vi "CT-Sweep One Component.vi"(0 "Phase In":dbl=100000.0, 5 "Last Freq (Hz)":dbl=100000.0, 7 "New Freq (Hz)":dbl=100000.0, 9 "dt (s)":dbl=100000.0, 11 "Npts":i32, 13 "randomize phase":bool) -> (4 "Phase Out":dbl, 8 "Y":dbl[](array[numeric]))   [LabVIEW 2015]
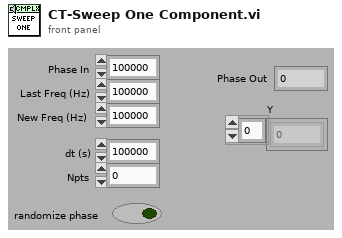
[diagram p1: front panel]
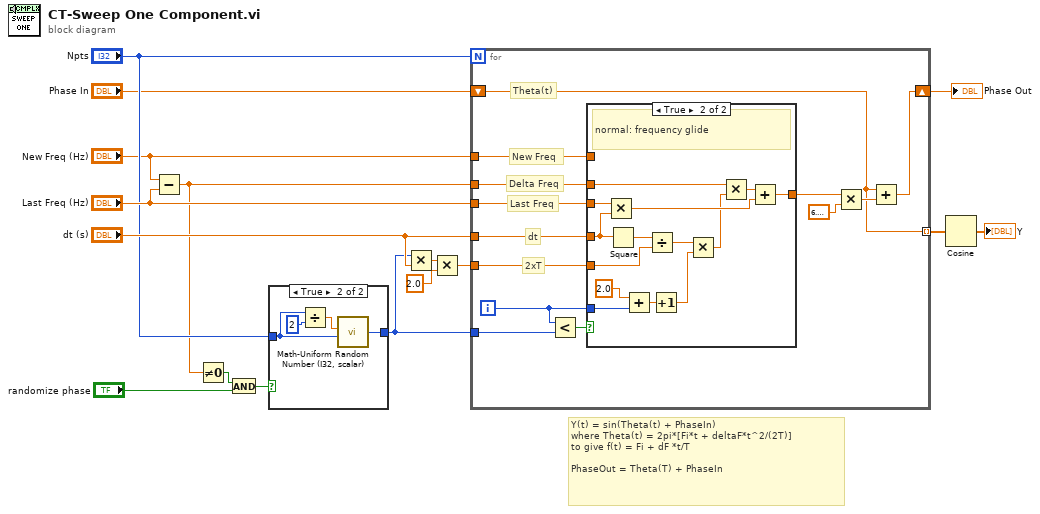
[diagram p0: block diagram]
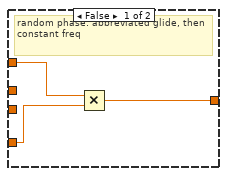
[diagram p3: hidden frame]
diagram:
  # "Y(t) = sin(Theta(t) + PhaseIn)\nwhere Theta(t) = 2pi*[Fi*t + deltaF*t^2/(2T)]\nto give f(t) = Fi + dF *t/T \n\nPhaseOut = Theta(T) + PhaseIn"
  n1 = Subtract(x="New Freq (Hz)", y="Last Freq (Hz)") -> (x-y=w6:dbl)
  n2 = Not Equal To 0?(x=w6) -> (x != 0?=w7:bool)
  n3 = And(x=w7, y="randomize phase") -> (x .and. y?=w3:bool)
  n4 = case shown="True" w3 {
    tunnel: "Npts" -> [w17 w20]
    tunnel: [w17 w18] -> w8
    frame False {
    }
    frame True {
      n5 = Divide(x=w20, y=2) -> (x/y=w19:dbl)
      n6 = call "Math-Uniform Random Number (I32, scalar).vi"("Ymax"=w20, "Ymin"=w19) -> ("Random Int"=w18:i32)  [unwired: 4 in]
    }
  }
  n7 = Multiply(x=w8, y="dt (s)") -> (x*y=w15:dbl)
  n8 = Multiply(x=w15, y=2.0) -> (x*y=w13:dbl)
  n9 = for {
    N: "Npts" -> [_]
    tunnel: "dt (s)" -> [w33]
    shift-right: [w29] -> w1
    shift-left: "Phase In" -> [w22]
    tunnel: "Last Freq (Hz)" -> [w34]
    tunnel: w13 -> [w27]
    tunnel: w6 -> [w28]
    tunnel: [w22] -> w4 mode=indexing
    tunnel: w8 -> [w25]
    tunnel: "New Freq (Hz)" -> [w24]
    i -> [w26]
    # "New Freq"
    # "dt"
    # "2xT"
    # "Theta(t)"
    # "Last Freq"
    # "Delta Freq"
    n10 = Less?(x=w26, y=w25) -> (x < y?=w23:bool)
    n11 = case shown="True" w23 {
      tunnel: w34 -> [_ w51]
      tunnel: w33 -> [w37 w50]
      tunnel: [w36 w45] -> w32
      tunnel: w28 -> [_ w44]
      tunnel: w27 -> [_ w43]
      tunnel: w26 -> [_ w41]
      tunnel: w24 -> [w35 _]
      frame False {
        # "random phase: abbreviated glide, then constant freq"
        n12 = Multiply(x=w35, y=w37) -> (x*y=w36:dbl)
      }
      frame True {
        # "normal: frequency glide"
        n13 = Multiply(x=w51, y=w50) -> (x*y=w46:dbl)
        n14 = Square(x=w50) -> (x^2=w49:dbl)
        n15 = Add(x=2.0, y=w41) -> (x+y=w39:dbl)
        n16 = Divide(x=w49, y=w43) -> (x/y=w48:dbl)
        n17 = Increment(x=w39) -> (x+1=w38:dbl)
        n18 = Multiply(x=w48, y=w38) -> (x*y=w42:dbl)
        n19 = Multiply(x=w44, y=w42) -> (x*y=w47:dbl)
        n20 = Add(x=w47, y=w46) -> (x+y=w45:dbl)
      }
    }
    n21 = Multiply(x=w32, y=6.283185307179586) -> (x*y=w30:dbl)
    n22 = Add(x=w22, y=w30) -> (x+y=w29:dbl)
  }
  "Phase Out" <- w1
  n23 = Cosine(x=w4) -> (cos(x)=→"Y":dbl[])
